vi "simple.vi"() -> (3 "Numeric":i32)   [LabVIEW 2011]
uses:
  myClass.lvclass
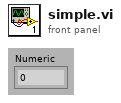
[diagram p1: front panel]
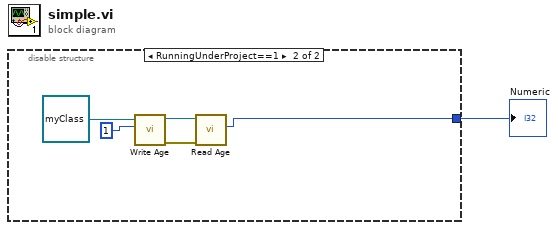
[diagram p0: block diagram]
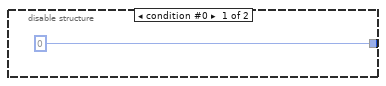
[diagram p2: hidden frame]
diagram:
  n1 = disable-structure shown="RunningUnderProject==1" {
    disable-tunnel: [0 w3] -> w1
    frame condition #0 {
    }
    frame condition #1 (active) {
      n2 = call-dynamic "Write Age.vi"("Age"=1 ("Numeric"), "myClass in"=refnum<class "myClass.lvclass"> refnum ("myClass.lvclass")) -> ("error out"=w4:errorcluster, "myClass out"=w5:refnum<class "myClass.lvclass">)  [unwired: 8 in]
      n3 = call-dynamic "Read Age.vi"("error in (no error)"=w4, "myClass in"=w5) -> ("Age"=w3:i32)  [unwired: 7 in, 2 out]
    }
  }
  "Numeric" <- w1
